vi "Set frame rate.vi"(8 "error in (no error)":errorcluster, 11 "DAQOrcaFlash in":refnum<class "DAQOrcaFlash.lvclass">) -> (0 "error out":errorcluster, 3 "DAQOrcaFlash out":refnum<class "DAQOrcaFlash.lvclass">)   [LabVIEW 2012, in "DAQOrcaFlash.lvclass"]
uses:
  DAQOrcaFlash.lvclass
  DAQOrcaFlash.lvclass/DAQOrcaFlash.ctl
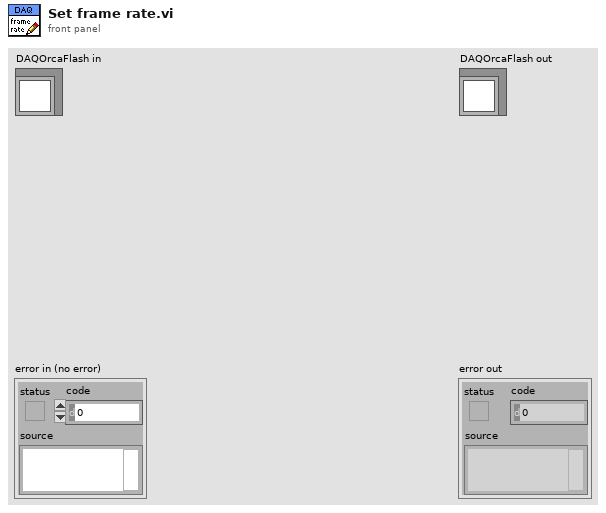
[diagram p1: front panel]
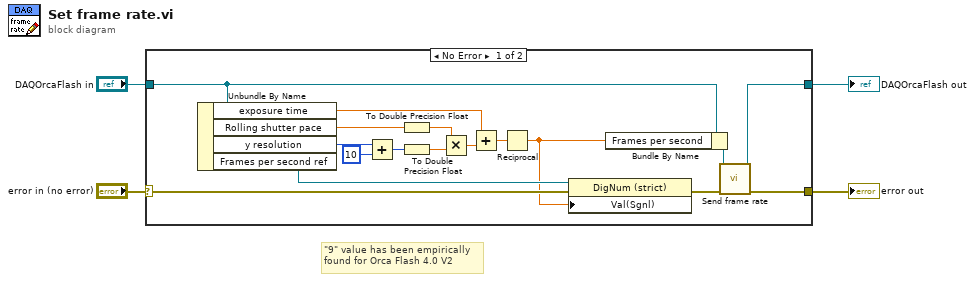
[diagram p0: block diagram]
diagram:
  # "\"9\" value has been empirically\nfound for Orca Flash 4.0 V2"
  n1 = case shown="No Error" "error in (no error)" {
    selector: "error in (no error)" -> [w13 w23]
    tunnel: [w7 w23] -> w3
    tunnel: [w5 w22] -> w1
    tunnel: "DAQOrcaFlash in" -> [w15 w22]
    frame No Error {
      n2 = Unbundle By Name(w15) -> ("exposure time"=w18:dbl[unit], "Rolling shutter pace"=w9:sgl[unit], "y resolution"=w21:i32, "Frames per second ref"=w14:refnum<vi>)
      n3 = Add(x=w21, y=10) -> (x+y=w19:i32)
      n4 = To Double Precision Float(number=w9) -> (double precision float=w10:dbl[unit])
      n5 = To Double Precision Float(number=w19) -> (double precision float=w11:dbl)
      n6 = Multiply(x=w10, y=w11) -> (x*y=w17:dbl[unit])
      n7 = Add(x=w18, y=w17) -> (x+y=w16:dbl[unit])
      n8 = Reciprocal(x=w16) -> (1/x=w12:dbl[unit])
      n9 = property class="DigNum (strict)"(reference=w14, error in=w13, "Val(Sgnl)"=w12) -> (error out=w8:errorcluster)  [unwired: 1 out]
      n10 = Bundle By Name(cluster=w15, "Frames per second"=w12) -> (w6:refnum<class "DAQOrcaFlash.lvclass">)
      n11 = call-dynamic "Send frame rate.vi"("error in (no error)"=w8, "DAQOrcaFlash in"=w6) -> ("error out"=w7:errorcluster, "DAQOrcaFlash out"=w5:refnum<class "DAQOrcaFlash.lvclass">)  [unwired: 8 in]
    }
    frame Error {
    }
  }
  "error out" <- w3
  "DAQOrcaFlash out" <- w1
